vi "myTask.vi"(8 "error in (no error)":errorcluster, 10 "stopMechanism":refnum<class "ITaskStopMechanism.lvclass">, 11 "ITask in":refnum<class "ITask.lvclass">) -> (0 "error out":errorcluster, 3 "ITask out":refnum<class "ITask.lvclass">)   [LabVIEW 2023, in "Task_BoolStopNotifier.lvclass"]
doc: "_____________________________________\nTLC Daemon 1.0.0.2\nCopyright (c) 2026 Andrea Cadei"
uses:
  Task_BoolStopNotifier.lvclass
  ITask/ITask.lvclass
  ITaskStopMechanism/ITaskStopMechanism.lvclass
  BoolNotifierStopMech/BoolNotifierStopMechanism.lvclass
  C:/projects/TLC_Daemon/.source/ITask/ITask.lvclass
  Task_BoolStopNotifier.lvclass/Task_BoolStopNotifier.ctl
  BoolNotifierStopMech/BoolNotifierStopMechanism.lvclass/BoolNotifierStopMechanism.ctl
  Write loopCounter.vi
  NotifierStopMechanism/Read notifierRef.vi
  Read description.vi
panel:
  out "loopCounter":i32 caption="Loop Counter"
  out "description":string
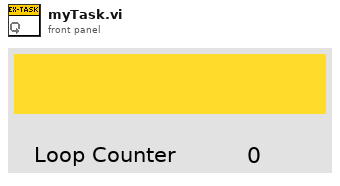
[diagram p1: front panel]
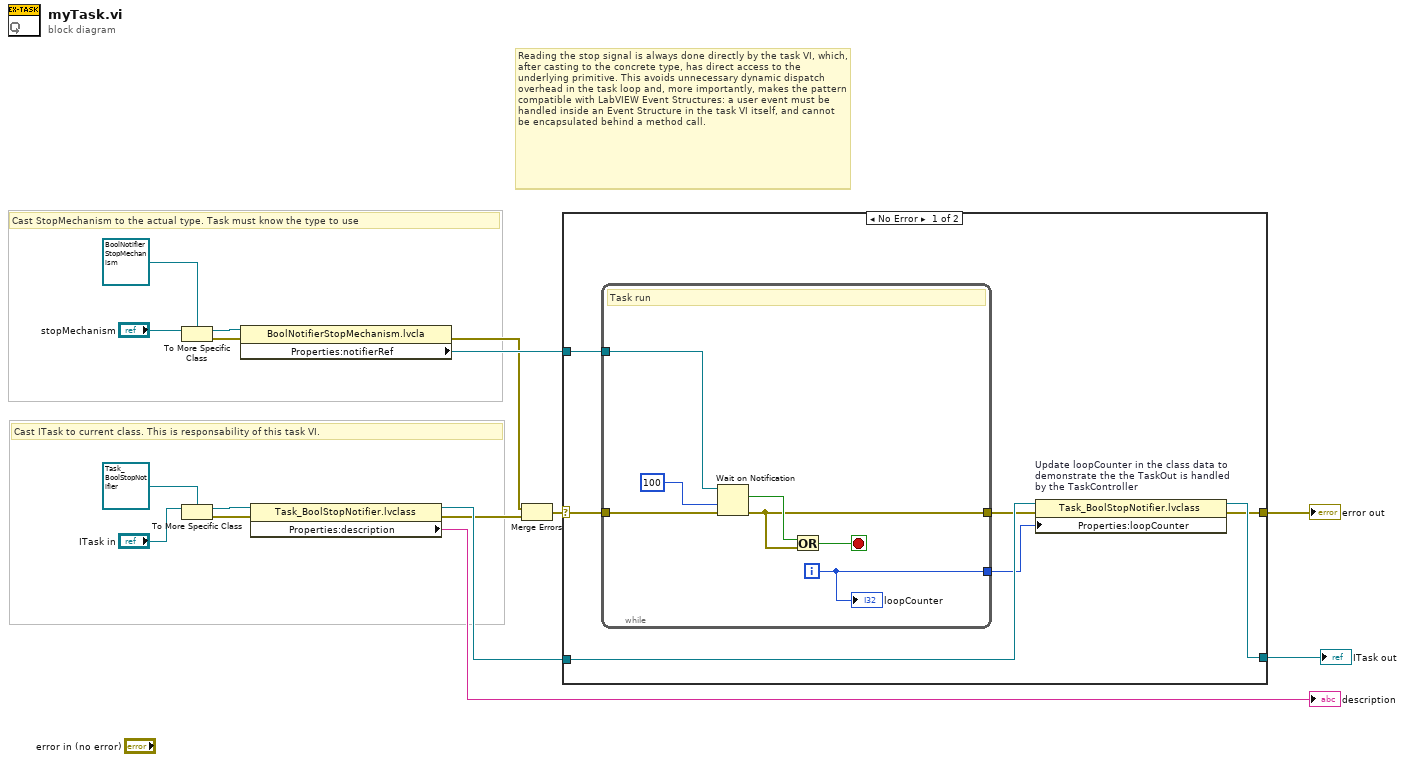
[diagram p0: block diagram]
diagram:
  # "Reading the stop signal is always done directly by the task VI, which, after casting to the concrete type, has direct access to the underlying primitive. This avoids unnecessary dynamic dispatch overhead in the task loop and, more importantly, makes the pattern compatible with LabVIEW Event Structures: a user event must be handled inside an Event Structure in the task VI itself, and cannot be encapsulated behind a method call."
  # "Reading the stop signal is always done directly by the task VI, which, after casting to the concrete type, has direct access to the underlying primitive. This avoids unnecessary dynamic dispatch overhead in the task loop and, more importantly, makes the pattern compatible with LabVIEW Event Structures: a user event must be handled inside an Event Structure in the task VI itself, and cannot be encapsulated behind a method call."
  # "Cast ITask to current class. This is responsability of this task VI."
  # "Cast StopMechanism to the actual type. Task must know the type to use"
  n1 = To More Specific Class(target class=refnum<class "BoolNotifierStopMechanism.lvclass"> refnum ("TLC_Daemon.lvlib:NotifierStopMechanism.lvclass"), reference="stopMechanism") -> (specific class reference=w9:refnum<class "BoolNotifierStopMechanism.lvclass">, error out=w5:errorcluster)  [unwired: 1 in]
  n2 = To More Specific Class(target class=refnum<class "Task_BoolStopNotifier.lvclass"> refnum ("ExampleTask_StopNotifier.lvclass"), reference="ITask in") -> (specific class reference=w11:refnum<class "Task_BoolStopNotifier.lvclass">, error out=w12:errorcluster)  [unwired: 1 in]
  n3 = property class="BoolNotifierStopMechanism.lvcla"(reference=w9, error in=w5) -> (error out=w3:errorcluster, "Properties:notifierRef"=w8:refnum<notifier>)  [unwired: 1 out]
  n4 = property class="Task_BoolStopNotifier.lvclass"(reference=w11, error in=w12) -> (reference out=w7:refnum<class "Task_BoolStopNotifier.lvclass">, error out=w4:errorcluster, "Properties:description"=→"description":string)
  n5 = Merge Errors(w3, w4) -> (w2:errorcluster)
  n6 = case shown="No Error" w2 {
    selector: w2 -> [w19 w32]
    tunnel: w8 -> [w23 _]
    tunnel: w7 -> [w22 w31]
    tunnel: [w20 w31] -> w6
    tunnel: [w17 w32] -> w1
    frame No Error {
      n7 = while {
        tunnel: w23 -> [w30]
        tunnel: w19 -> [w26]
        tunnel: [w25] -> w18
        tunnel: [w24] -> w21
        i -> [w24]
        stop <- w27 stop-if-true
        # "Task run"
        n8 = Wait on Notification(notifier=w30, timeout in ms (-1)=100, error in (no error)=w26) -> (notification=w28:bool, error out=w25:errorcluster)  [unwired: 1 in, 2 out]
        n9 = Or(x=w28, y=w25) -> (x .or. y?=w27:bool)
        "loopCounter" <- w24
      }
      n10 = property on="Update loopCounter in the class data to\ndemonstrate the the TaskOut is handled\nby the TaskController" class="Task_BoolStopNotifier.lvclass"(reference=w22, error in=w18, "Properties:loopCounter"=w21) -> (reference out=w20:refnum<class "Task_BoolStopNotifier.lvclass">, error out=w17:errorcluster)
    }
    frame Error {
    }
  }
  "error out" <- w1
  "ITask out" <- w6
